vi "ICNC Connect.vi"(8 "error in (no error)":errorcluster caption="entrée d'erreur (pas d'erreur)", 11 "ICNC_Number":u32) -> (0 "error out":errorcluster caption="sortie d'erreur", 3 "function return":u32)   [LabVIEW 2017, in "ICNC2.lvlib"]
doc: "DWORD ICNC_Connect( DWORD ICNC_Number=0);"
uses:
  <userlib>/ICNC/ICNC2.lvlib
  <userlib>/ICNC/ICNC2.dll
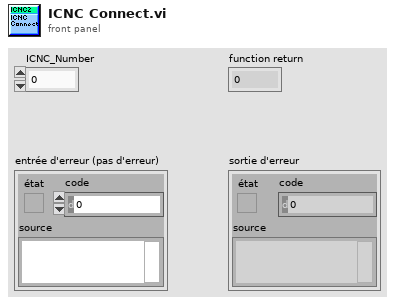
[diagram p1: front panel]
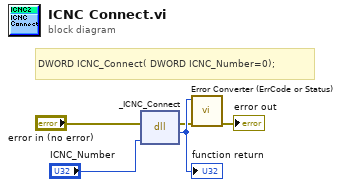
[diagram p0: block diagram]
diagram:
  # "DWORD ICNC_Connect( DWORD ICNC_Number=0);"
  n1 = dll-call lib="C:/Program Files (x86)/National Instruments/LabVIEW 2017/user.lib/ICNC/ICNC2.*" fn="_ICNC_Connect"(error in="error in (no error)", "ICNC_Number"="ICNC_Number") -> (error out=w2:errorcluster, w5:u32)  [unwired: 3 in, 1 out]
  "function return" <- w5
  n2 = call <userlib>:"Error Converter (ErrCode or Status).vi"("error in (no error)"=w2, "error code"=w5) -> ("error out"=→"error out":errorcluster)  [unwired: 9 in]
